vi "serail_testv2.1.vi"() -> ()   [LabVIEW 2016]
uses:
  <vilib>/Instr/_visa.llb/VISA Configure Serial Port (Instr).vi
panel:
  out "Yazılan":string
  out "x/y":dbl
  in  "Teta Aralık":dbl=10.0
  out "i":i32
  in  "Numeric Control":i32=260
  in  "Motor Driver Port":refnum<visa-resource-name>="COM5"
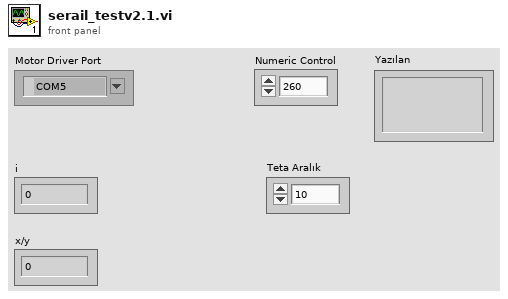
[diagram p1: front panel]
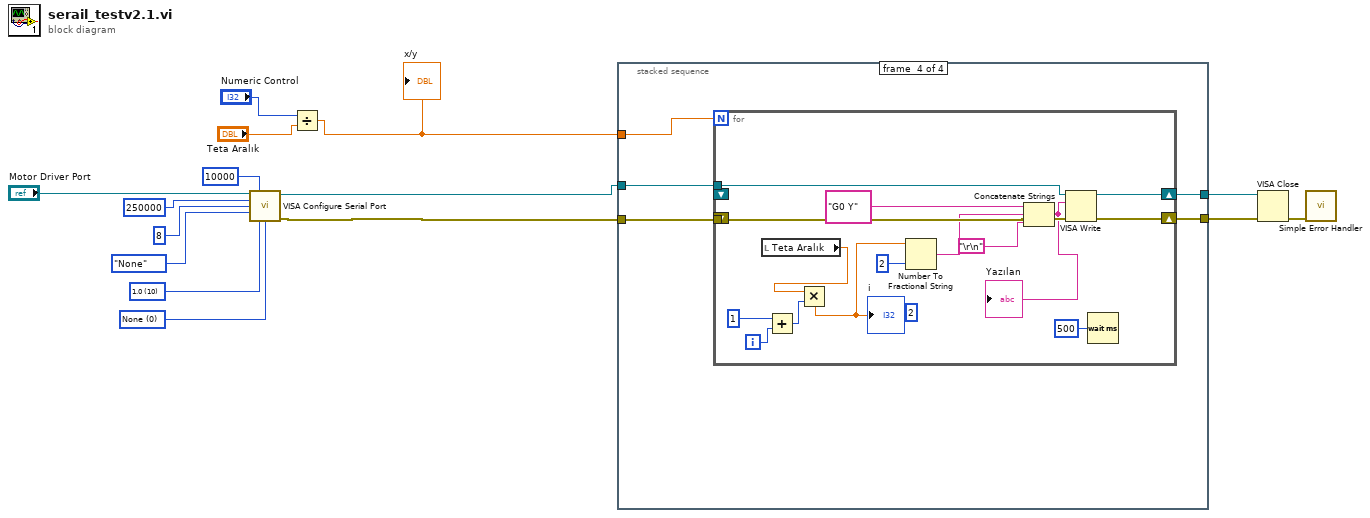
[diagram p0: block diagram]
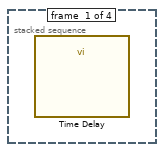
[diagram p2: hidden frame]
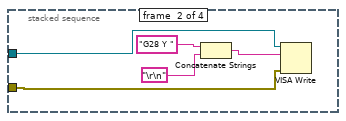
[diagram p3: hidden frame]
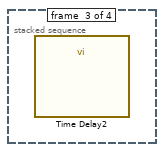
[diagram p4: hidden frame]
diagram:
  w9 = u16 0 items=["None", "XON/XOFF", "RTS/CTS", "XON/XOFF & RTS/CTS", "DTR/DSR", "XON/XOFF & DTR/DSR"] ("flow control (0:none)")
  w10 = u16 10 items=["1.0"=10, "1.5"=15, "2.0"=20] ("stop bits (10: 1 bit)")
  n1 = call-poly "VISA Configure Serial Port"("VISA resource name"="Motor Driver Port", "timeout (10sec)"=u32 10000, "baud rate (9600)"=u32 250000, "data bits (8)"=u16 8, "parity (0:none)"=enum16{"None", "Odd", "Even", "Mark", "Space"}."None", "stop bits (10: 1 bit)"=w10, "flow control (0:none)"=w9) -> ("VISA resource name out"=w1:refnum<visa-resource-name>, "error out"=w2:errorcluster)  [unwired: 7 in]
  n2 = Divide(x="Numeric Control", y="Teta Aralık") -> (x/y=w4:dbl)
  "x/y" <- w4
  n3 = stacked-sequence {
    tunnel: [_ _ _ w25] -> w7
    tunnel: [_ _ _ w24] -> w3
    tunnel: w4 -> [_ _ _ w23]
    tunnel: w1 -> [_ w17 _ w22]
    tunnel: w2 -> [_ w16 _ w21]
    frame #0 {
      n4 = call "Time Delay"() -> ()  [unwired: 11 in, 1 out]
    }
    frame #1 {
      n5 = Concatenate Strings("G28 Y " ("write buffer"), "\r\n") -> (w18:string)
      n6 = VISA Write(VISA resource name=w17, write buffer=w18, error in (no error)=w16) -> ()  [unwired: 3 out]
    }
    frame #2 {
      n7 = call "Time Delay2"() -> ()  [unwired: 11 in, 1 out]
    }
    frame #3 {
      n8 = for {
        N: w23 -> [_]
        tunnel: w22 -> [w40]
        tunnel: w21 -> [w39]
        shift-right: [w37] -> w25
        shift-left: _ -> [_]
        shift-right: [w38] -> w24
        shift-left: _ -> [_]
        i -> [w32]
        (unwired) i16 2 ("precision (6)")
        n9 = local read "Teta Aralık"() -> (w30:dbl)
        n10 = Add(x=1, y=w32) -> (x+y=w29:i32)
        n11 = Multiply(x=w30, y=w29) -> (x*y=w26:dbl)
        "i" <- w26
        n12 = Number To Fractional String(number=w26, precision (6)=i16 2) -> (F-format string=w27:string)  [unwired: 2 in]
        n13 = Concatenate Strings("G0 Y" ("string"), w27, "\r\n") -> (w36:string)
        "Yazılan" <- w36
        n14 = VISA Write(VISA resource name=w40, write buffer=w36, error in (no error)=w39) -> (VISA resource name out=w37:refnum<visa-resource-name>, error out=w38:errorcluster)  [unwired: 1 out]
        n15 = Wait (ms)(milliseconds to wait=u32 500) -> ()  [unwired: 1 out]
      }
    }
  }
  n16 = VISA Close(VISA resource name=w7, error in (no error)=w3) -> (error out=w8:errorcluster)
  n17 = call <vilib>:"Simple Error Handler.vi"("error in (no error)"=w8) -> ()  [unwired: 4 in, 5 out]
